vi "advance array manipulation part2.vi"() -> ()   [LabVIEW 2016]
panel:
  out "Output Array":dbl[][](array[numeric])
  in  "Dimention-Column":i32
  in  "Dimention-Row":i32
  in  "Input Array":dbl[](array[numeric])
  out "Minimum Index":i32[](array[numeric])
  out "Minimum Value":dbl
  out "Maximum Index":i32[](array[numeric])
  out "Maximum Value":dbl
  in  "Input Array":dbl[][](array[numeric])
  out "Subset Array":dbl[](array[numeric])
  in  "Length":i32
  in  "Index":i32
  in  "Input Array":dbl[](array[numeric])
  out "Appended Array":dbl[][](array[numeric])
  in  "Array3":dbl[](array[numeric])
  in  "Array2":dbl[](array[numeric])
  in  "Array1":dbl[](array[numeric])
  out "Ooutput Array":dbl[][](array[numeric])
  in  "Element":dbl
  in  "Dimention Column":i32
  in  "Dimontion Row":i32
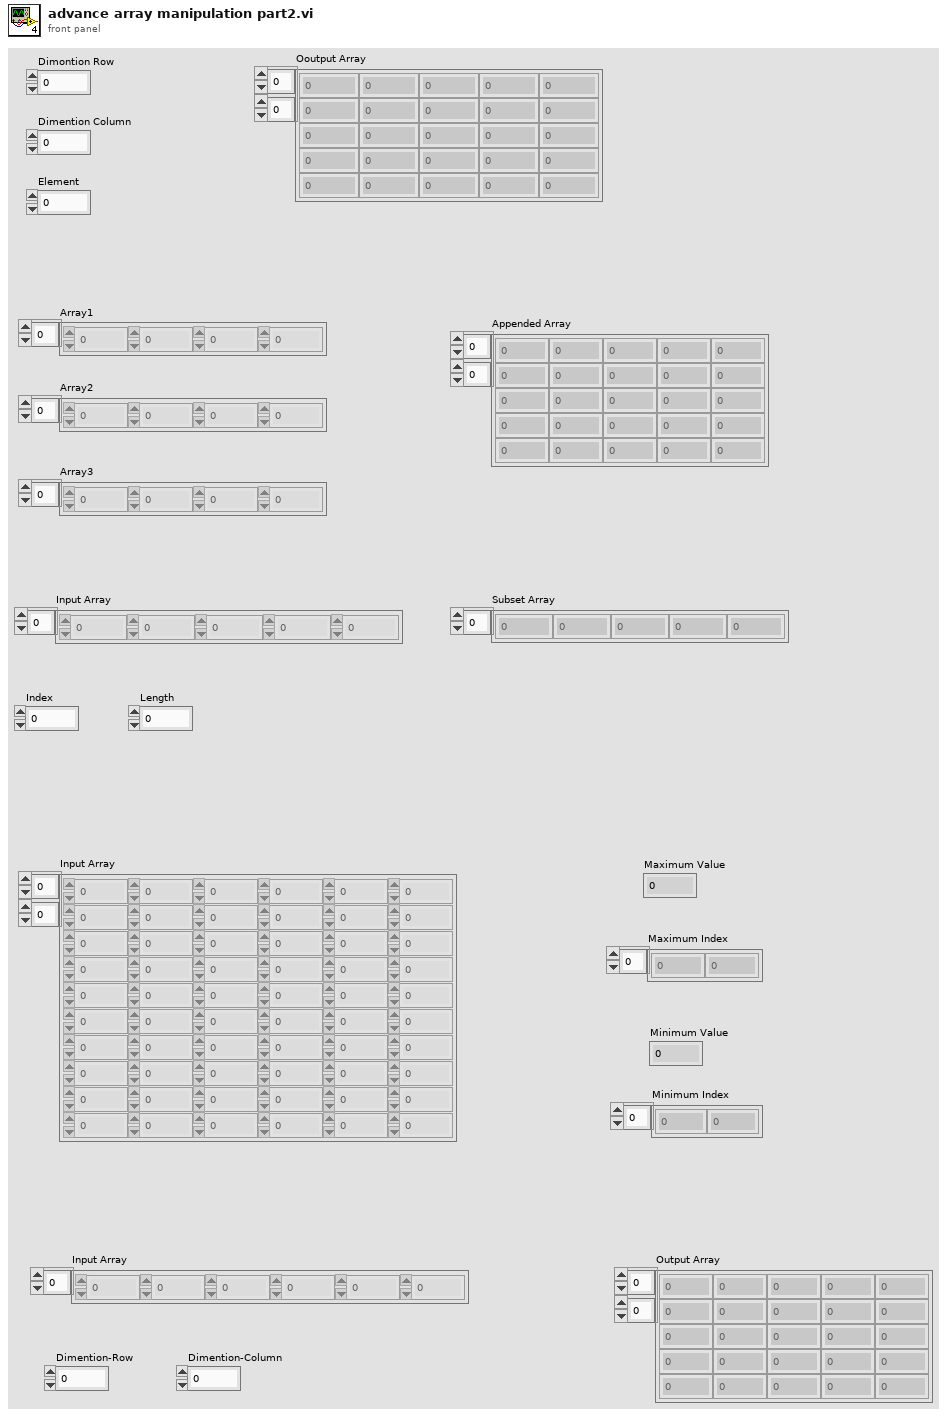
[diagram p1: front panel]
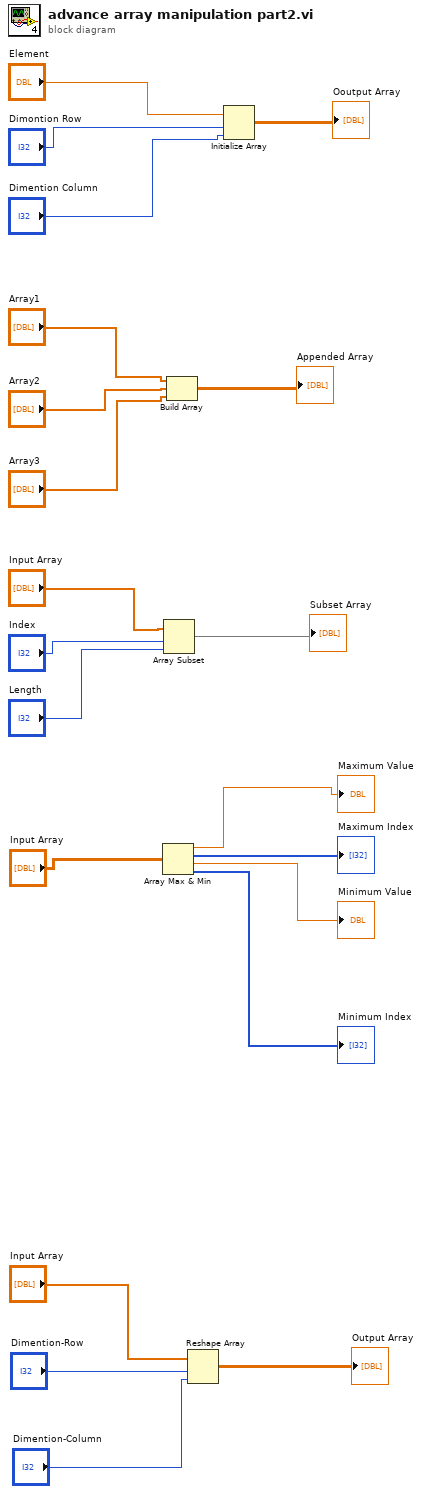
[diagram p0: block diagram]
diagram:
  n1 = Array Max & Min(array="Input Array") -> (max value=→"Maximum Value":dbl, max index (indices)=→"Maximum Index":i32[], min value=→"Minimum Value":dbl, min index (indices)=→"Minimum Index":i32[])
  n2 = Array Subset(array="Input Array", index="Index", length="Length") -> (→"Subset Array":dbl[])
  n3 = Build Array("Array1", "Array2", "Array3") -> (→"Appended Array":dbl[][])
  n4 = Reshape Array("Input Array", "Dimention-Row", "Dimention-Column") -> (→"Output Array":dbl[][])
  n5 = Initialize Array("Element", "Dimontion Row", "Dimention Column") -> (→"Ooutput Array":dbl[][])
